vi "PH_BackreflectionMeas.establish connection.vi"(0 "i ref in":refnum<vi>, 5 "error in":errorcluster) -> (14 "i ref out":refnum<vi>, 19 "error out":errorcluster)   [LabVIEW 2014, in "PH_BackreflectionMeas.lvlib"]
doc: "This VI checks the connection and resets the hardware."
uses:
  PH_BackreflectionMeas.lvlib
  PH_TKTDS-30xx/PH_TKTDS-30xx.lvlib
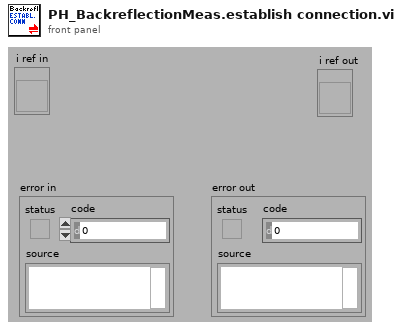
[diagram p1: front panel]
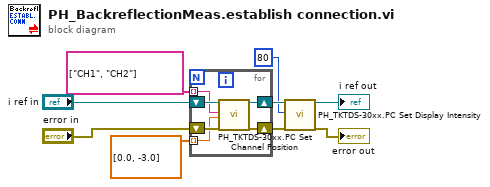
[diagram p0: block diagram]
diagram:
  n1 = for {
    shift-right: [w12] -> w9
    shift-left: "i ref in" -> [w13]
    shift-right: [w14] -> w8
    shift-left: "error in" -> [w15]
    tunnel: string[] ["CH1", "CH2"] -> [w11] mode=indexing
    tunnel: dbl[] [0.0, -3.0] -> [w10] mode=indexing
    n2 = call "PH_TKTDS-30xx.PC Set Channel Position.vi"("i ref in"=w13, "Channel Name"=w11, "Position (0)"=w10, "error IO"=w15) -> ("i ref out"=w12:refnum<vi>, "error out"=w14:errorcluster)  [unwired: 14 in]
  }
  n3 = call "PH_TKTDS-30xx.PC Set Display Intensity.vi"("i ref in"=w9, "Intensity (1)"=u8 80, "error IO"=w8) -> ("i ref out"=→"i ref out":refnum<vi>, "error out"=→"error out":errorcluster)  [unwired: 15 in]
